vi "纳清DO_第一点原始数据写入.vi"(8 "error in (no error)":errorcluster caption="错误输入（无错误）", 10 "数值":sgl, 11 "MB session in":refnum<class "MB_Master.lvclass">) -> (0 "error out":errorcluster caption="错误输出", 3 "MB session out":refnum<class "MB_Master.lvclass">)   [LabVIEW 2016, in "斯坦道多参数.lvlib"]
uses:
  <vilib>/Plasmionique/MB Master/MB_Master/MB_Master.lvclass
  <vilib>/Plasmionique/MB Master/MB Master.lvlib
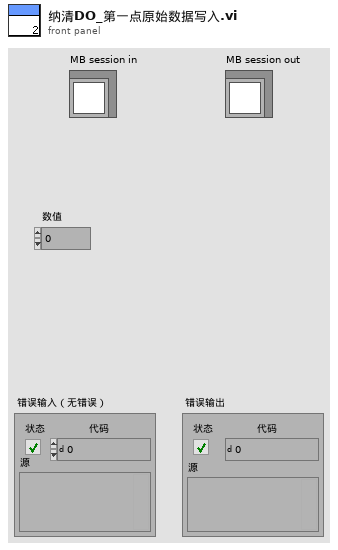
[diagram p1: front panel]
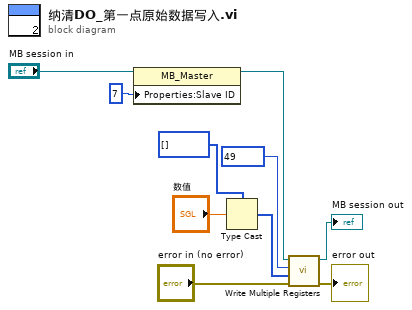
[diagram p0: block diagram]
diagram:
  n1 = property class="MB_Master"(reference="MB session in", "Properties:Slave ID"=u8 7 ("Slave ID")) -> (reference out=w7:refnum<class "MB_Master.lvclass">)  [unwired: 1 in, 1 out]
  n2 = Type Cast(type=u16[] [], x="数值") -> (*(type *) &x=w1:u16[])
  n3 = call <vilib>:"Write Multiple Registers.vi"("error in (no error)"="error in (no error)", "values"=w1, "starting address"=u16 49, "MB session in"=w7) -> ("error out"=→"error out":errorcluster, "MB session out"=→"MB session out":refnum<class "MB_Master.lvclass">)  [unwired: 6 in]
